vi "2 Global Old Version for Jason's Benefit.vi"() -> ()   [LabVIEW 2011]
panel:
  in  "Rudder Angle":dbl
  in  "Perceived Wind":cluster{"X Position":dbl, "Y Position":dbl}
  in  "Robot Velocity":cluster{"X Position":dbl, "Y Position":dbl}
  in  "Robot Location":cluster{"X Position":dbl, "Y Position":dbl}
  # "All distances in meters\nAll angles in radians\nAll speeds in meters per second\nX-Y make a right handed coordinate system with Z pointing up\nPositive Rudder angle makes the boat turn right\nX-Y Coordinates are based on GPS and are in a global frame"
  # "Sense Abstractions / Inputs from Simulation"
  # "Act Abstractions / Outputs to Simulation"
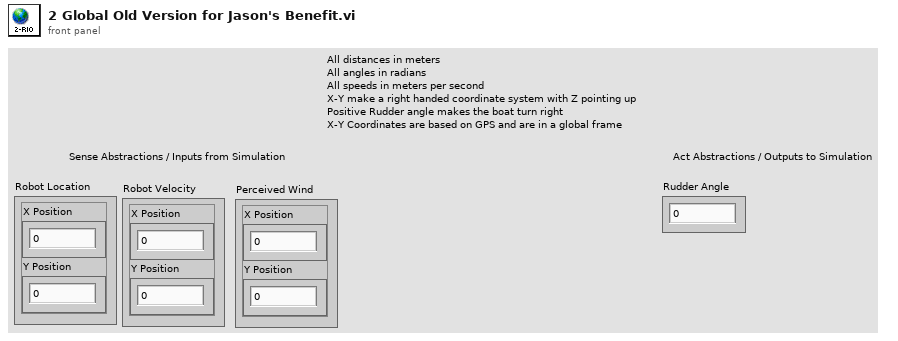
[diagram p1: front panel]
diagram:
